vi "Calc Mean.vi"(11 "JSON Value In":refnum<class "JSON Value.lvclass">) -> (3 "JSON Value":refnum<class "JSON Value.lvclass">)   [LabVIEW 2020, in "Library Commun.lvlib" / "JSON Value.lvclass"]
uses:
  JSON Value.lvclass
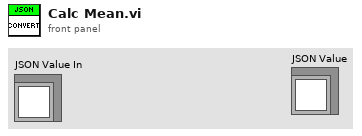
[diagram p1: front panel]
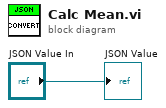
[diagram p0: block diagram]
diagram:
  "JSON Value" <- "JSON Value In"
